vi "SwerveWheel.vi"(9 "rotate only?":bool, 10 "Inputs":dbl[](array[numeric]), 11 "Wheel":T1(ring)) -> (2 "Angle":dbl, 3 "Speed":dbl)   [LabVIEW 2019]
uses:
  <vilib>/Rock Robotics/WPI/ThirdParty/Phoenix-LabVIEW/Motor Controller/Controls/CTRE_Phoenix_MotorControl_ControlMode.ctl
  <vilib>/Analysis/coordinate.llb/Angle Range (Degree).ctl
  <vilib>/Analysis/coordinate.llb/Angle Units.ctl
  <vilib>/Analysis/coordinate.llb/Wrap Angle (scalar).vi
  Robot Global Data.vi
  <vilib>/Rock Robotics/WPI/ThirdParty/Phoenix-LabVIEW/Motor Controller/Get/CTRE_Phoenix_MotorController_IntegratedSensorData_TalonFX.vi
  <vilib>/Analysis/NI_AAL_Angle.lvlib
  <vilib>/Rock Robotics/WPI/ThirdParty/Phoenix-LabVIEW/Motor Controller/Controls/CTRE_Phoenix_MotorControl_TalonFXInvertType.ctl
  <vilib>/Rock Robotics/WPI/ThirdParty/Phoenix-LabVIEW/Motor Controller/Get/CTRE_Phoenix_MotorController_GetSupplyAndStatorCurrent_Enhanced.vi
  <vilib>/Rock Robotics/WPI/ThirdParty/Phoenix-LabVIEW/Motor Controller/Get/CTRE_Phoenix_MotorController_GetGeneralStatus.vi
panel:
  out "Z":bool
  out "Distance 2":dbl
  out "Distance":dbl
  out "Current Pos":dbl format="%.2f"
  out "Position to go to":dbl
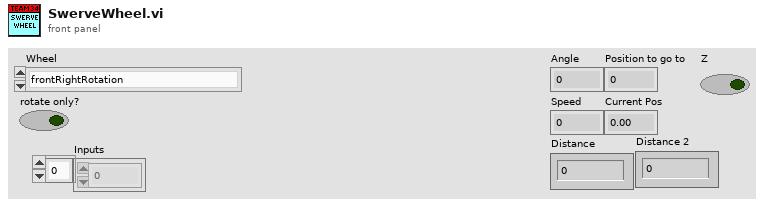
[diagram p1: front panel]
types:
  T1 = enum16{"frontRightRotation", "frontLeftRotation", "backRightRotation", "backLeftRotation"}
  T2 = typedef "NI_AAL_Angle.lvlib/Angle Units.ctl" = i32
  T3 = typedef "NI_AAL_Angle.lvlib/Angle Range (Degree).ctl" = u16
  T4 = typedef "CTRE_Phoenix_MotorControl_ControlMode.ctl" = u16
  T5 = typedef "CTRE_Phoenix_MotorControl_TalonFXInvertType.ctl" = enum16{"Counter-Clockwise", "Clockwise"}
  T6 = typedef "WPI_MotorControlDeviceRef.ctl" = cluster{"DeviceStatus":errorcluster, "Type":T7, "PWM":cluster{"PWM Channel":T8, "DeadBand":T9}, "CAN":cluster{"Device Number":u8, "SetOutput VI Ref":variant, "GetOutput VI Ref":variant, "Enable VI Ref":variant, "Disable VI Ref":variant, "Data":variant}, "Invert":bool, "DIO PWM":cluster{"PWM \"Enable\" Channel":T8, "DIOChannel":T10, "PWM Rate":dbl}}
  T7 = typedef "WPI_MotorControlType.ctl" = enum16{"PWM", "CAN", "DIO PWM"}
  T8 = typedef "FPGA_DIOPWMChannel.ctl" = enum8{"PWM 0", "PWM 1", "PWM 2", "PWM 3", "PWM 4", "PWM 5", "PWM 6", "PWM 7", "PWM 8", "PWM 9", "PWM MXP 0", "PWM MXP 1", "PWM MXP 2", "PWM MXP 3", "PWM MXP 4", "PWM MXP 5", "PWM MXP 6", "PWM MXP 7", "PWM MXP 8", "PWM MXP 9", "Invalid"}
  T9 = typedef "WPI_PWMDeadband.ctl" = cluster{"Name":string, "maxPositivePwm":i32, "minPositivePwm":i32, "centerPwm":i32, "maxNegativePwm":i32, "minNegativePwm":i32, "angularRange":u16}
  T10 = typedef "FPGA_DIOChannel.ctl" = enum8{"DIO 0", "DIO 1", "DIO 2", "DIO 3", "DIO 4", "DIO 5", "DIO 6", "DIO 7", "DIO 8", "DIO 9", "DIO MXP 0", "DIO MXP 1", "DIO MXP 2", "DIO MXP 3", "DIO MXP 4", "DIO MXP 5", "DIO MXP 6", "DIO MXP 7", "DIO MXP 8", "DIO MXP 9", "DIO MXP 10", "DIO MXP 11", "DIO MXP 12", "DIO MXP 13", "DIO MXP 14", "DIO MXP 15", "SPI Port CS1", "SPI Port CS2", "SPI Port CS3", "SPI Port MISO", "SPI Port MOSI", "Invalid"}
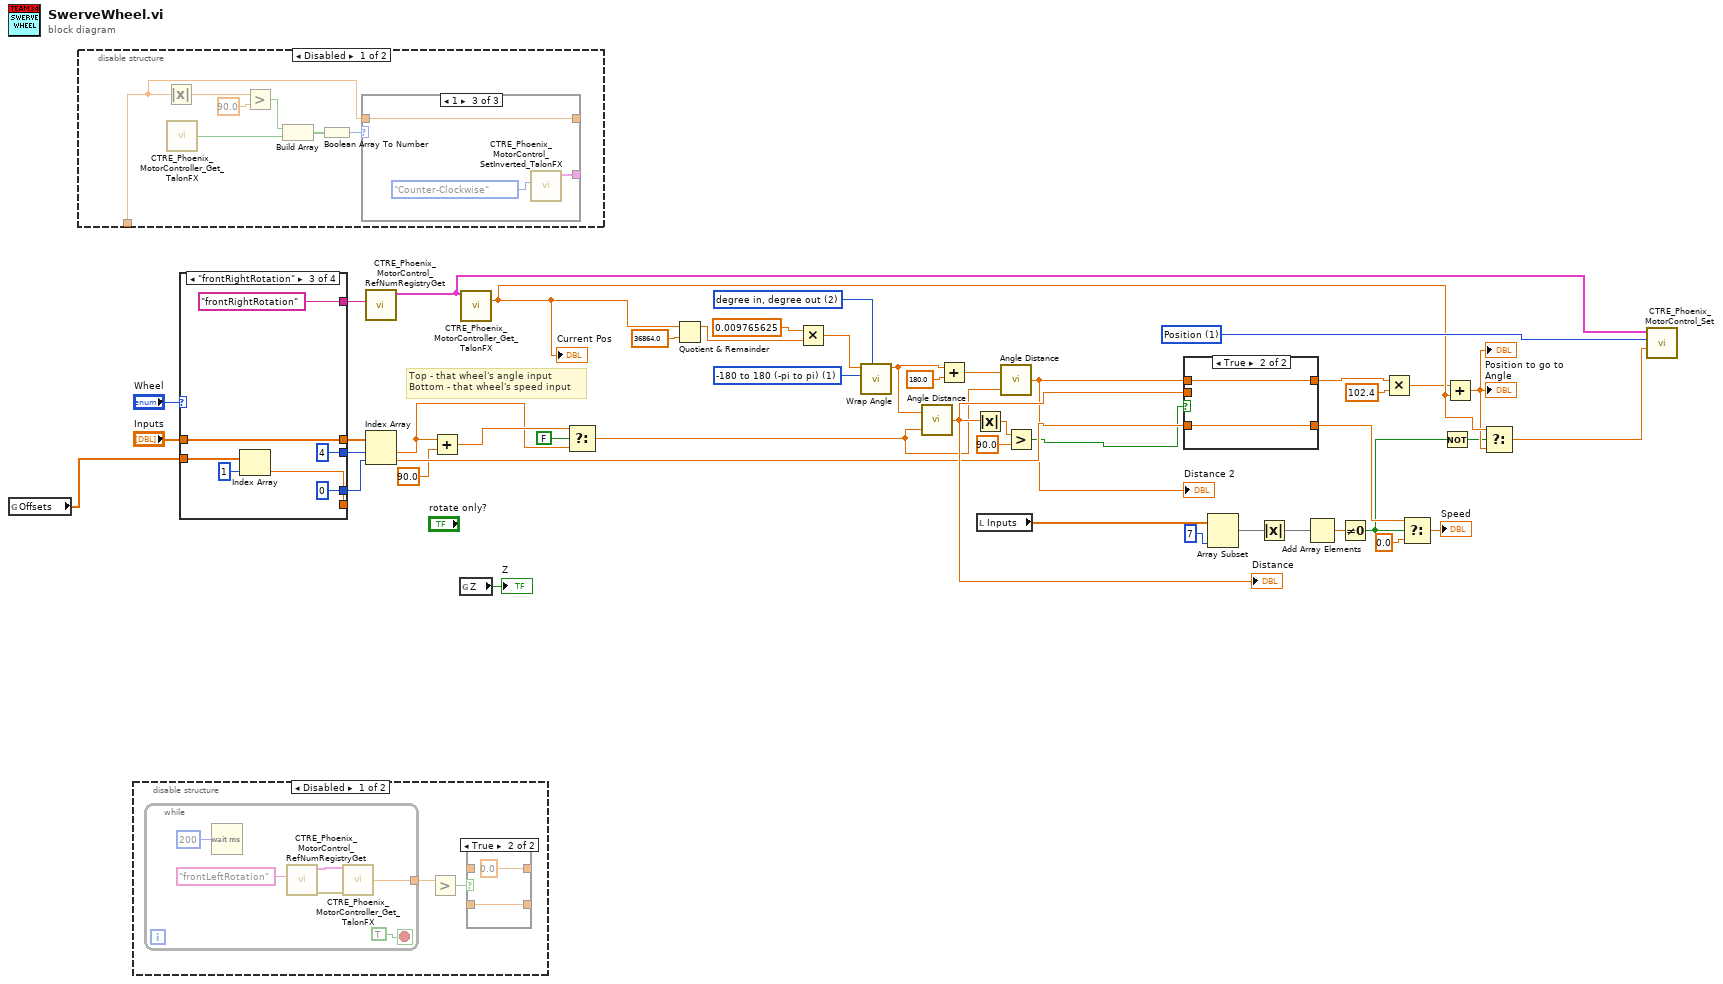
[diagram p0: block diagram]
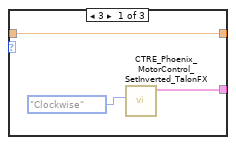
[diagram p2: hidden frame]
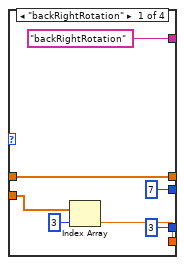
[diagram p5: hidden frame]
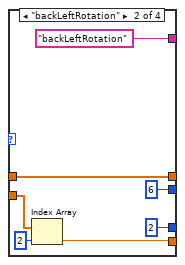
[diagram p6: hidden frame]
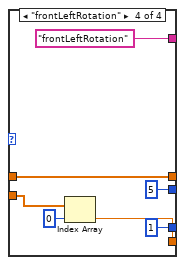
[diagram p7: hidden frame]
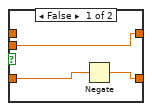
[diagram p10: hidden frame]
diagram:
  w43 = T2 2 items=["radian in, radian out", "radian in, degree out", "degree in, degree out", "degree in, radian out"] ("angle units")
  w44 = T3 1 items=["none", "-180 to 180 (-pi to pi)", "0 to 360 (0 to 2pi)"] ("angle range")
  w45 = T4 1 items=["PercentOutput"=0, "Position"=1, "Velocity"=2, "Current"=3, "Follower"=5, "MotionProfile"=6, "MotionMagic"=7, "MotionProfileArc"=10, "Disabled"=15] ("Control Mode")
  # "Top - that wheel's angle input\nBottom - that wheel's speed input"
  n1 = global read "Robot Global Data.vi" "Offsets"() -> (w10:dbl[])
  n2 = disable-structure shown="Disabled" {
    disable-tunnel: _ -> [w53 _]
    frame Disabled {
      n3 = Absolute Value(x=w53) -> (abs(x)=w52:dbl)
      n4 = call-poly <vilib>:"CTRE_Phoenix_MotorController_Get_TalonFX.vi"() -> ("Inverted?"=w49:bool)  [unwired: 10 in, 5 out]
      n5 = Greater?(x=w52, y=90.0) -> (0:w50:bool)
      n6 = Build Array(w50, w49) -> (w48:bool[])
      n7 = Boolean Array To Number(Boolean array=w48) -> (number=w47:u32)
      n8 = case shown="1" w47 {
        tunnel: w53 -> [w55 w57 w59]
        tunnel: [w55 w57 w59] -> _
        tunnel: [w54 _ w58] -> _
        frame 3 {
          n9 = call <vilib>:"CTRE_Phoenix_MotorControl_SetInverted_TalonFX.vi"("Invert Type"=CTRE_Phoenix_MotorControl_TalonFXInvertType."Clockwise") -> ("PhoenixMotorControlDevRef"=w54:T6)  [unwired: 9 in, 1 out]
        }
        frame 0, Default {
        }
        frame 1 {
          n10 = call <vilib>:"CTRE_Phoenix_MotorControl_SetInverted_TalonFX.vi"("Invert Type"=CTRE_Phoenix_MotorControl_TalonFXInvertType."Counter-Clockwise") -> ("PhoenixMotorControlDevRef"=w58:T6)  [unwired: 9 in, 1 out]
        }
      }
    }
    frame Enabled {
    }
  }
  n11 = disable-structure shown="Disabled" {
    frame Disabled {
      n12 = while {
        tunnel: [w67] -> w62
        stop <- TRUE stop-if-true
        n13 = Wait (ms)(milliseconds to wait=u32 200) -> ()  [unwired: 1 out]
        n14 = call <vilib>:"CTRE_Phoenix_MotorControl_RefNumRegistryGet.vi"("refnum name"="frontLeftRotation") -> ("error out"=w69:errorcluster, "PhoenixMotorControlDevRef"=w70:T6)  [unwired: 9 in]
        n15 = call-poly <vilib>:"CTRE_Phoenix_MotorController_Get_TalonFX.vi"("PhoenixMotorControlDevRef"=w70, "error in"=w69) -> ("Stator Current"=w67:dbl)  [unwired: 10 in, 3 out]
      }
      n16 = Greater?(x=w62) -> (0:w61:bool)  [unwired: 1 in]
      n17 = case shown="True" w61 {
        tunnel: [w64 0.0] -> _
        tunnel: _ -> [w64 _]
        tunnel: [w63 w66] -> _
        tunnel: _ -> [w63 w66]
        frame False {
        }
        frame True {
        }
      }
    }
    frame Enabled {
    }
  }
  n18 = case shown="\"frontRightRotation\"" "Wheel" {
    tunnel: ["backRightRotation" "backLeftRotation" "frontRightRotation" "frontLeftRotation"] -> w46
    tunnel: [3 ("index") 2 ("index") 0 ("index") 1 ("index")] -> w24
    tunnel: [7 ("index") 6 ("index") 4 ("index") 5 ("index")] -> w23
    tunnel: "Inputs" -> [w79 w86 w92 w97]
    tunnel: [w79 w86 w92 w97] -> w14
    tunnel: w10 -> [w75 w82 w89 w96]
    tunnel: [w74 w81 w88 w95] -> _
    frame "backRightRotation" {
      n19 = Index Array(array=w75, index=3) -> (element=w74:dbl)
    }
    frame "backLeftRotation" {
      n20 = Index Array(array=w82, index=2) -> (element=w81:dbl)
    }
    frame "frontRightRotation" {
      n21 = Index Array(array=w89, index=1) -> (element=w88:dbl)
    }
    frame "frontLeftRotation" {
      n22 = Index Array(array=w96, index=0) -> (element=w95:dbl)
    }
  }
  n23 = call <vilib>:"CTRE_Phoenix_MotorControl_RefNumRegistryGet.vi"("refnum name"=w46) -> ("PhoenixMotorControlDevRef"=w3:T6)  [unwired: 9 in, 1 out]
  n24 = Index Array(array=w14, index #1=w23, index #2=w24) -> (element #1=w5:dbl, element #2=w29:dbl)
  n25 = Add(x=w5, y=90.0) -> (x+y=w7:dbl)
  n26 = global read "Robot Global Data.vi" "Z"() -> (→"Z":bool)
  n27 = call-poly <vilib>:"CTRE_Phoenix_MotorController_Get_TalonFX.vi"("PhoenixMotorControlDevRef"=w3) -> ("Position"=w21:dbl)  [unwired: 10 in, 4 out]
  "Current Pos" <- w21
  n28 = Select(t=w7, s=FALSE, f=w5) -> (s? t:f=w6:dbl)
  n29 = Quotient & Remainder(x=w21, y=36864.0) -> (x-y*floor(x/y)=w26:dbl)  [unwired: 1 out]
  n30 = Multiply(x=0.009765625, y=w26) -> (x*y=w25:dbl)
  n31 = call-poly <vilib>:"Wrap Angle.vi"("angle units"=w43, "angle range"=w44, "angle in"=w25) -> ("angle out"=w40:dbl)  [unwired: 7 in, 1 out]
  n32 = call "Angle Distance.vi"("Target Angle"=w6, "Current Angle"=w40) -> ("Distance"=w39:dbl)
  "Distance" <- w39
  n33 = Add(x=w40, y=180.0) -> (x+y=w41:dbl)
  n34 = Absolute Value(x=w39) -> (abs(x)=w38:dbl)
  n35 = local read "Inputs"() -> (w31:dbl[])
  n36 = call "Angle Distance.vi"("Target Angle"=w6, "Current Angle"=w41) -> ("Distance"=w22:dbl)
  "Distance 2" <- w22
  n37 = Greater?(x=w38, y=90.0) -> (0:w8:bool)
  n38 = case shown="True" w8 {
    tunnel: w39 -> [w103 _]
    tunnel: w22 -> [_ w105]
    tunnel: [w102 w104] -> w19
    tunnel: [w103 w105] -> w2
    tunnel: w29 -> [w101 w104]
    frame False {
      n39 = Negate(x=w101) -> (-x=w102:dbl)
    }
    frame True {
    }
  }
  n40 = Array Subset(array=w31, length=7) -> (w33:dbl[])  [unwired: 1 in]
  n41 = Absolute Value(x=w33) -> (abs(x)=w34:dbl[])
  n42 = Add Array Elements(numeric array=w34) -> (sum=w32:dbl)
  n43 = Not Equal To 0?(x=w32) -> (x != 0?=w17:bool)
  n44 = Multiply(x=w2, y=102.4) -> (x*y=w11:dbl)
  n45 = Select(t=w19, s=w17, f=0.0) -> (s? t:f=→"Speed":dbl)
  n46 = Not(x=w17) -> (.not. x?=w18:bool)
  n47 = Add(x=w11, y=w21) -> (x+y=w20:dbl)
  "Angle" <- w20
  "Position to go to" <- w20
  n48 = Select(t=w21, s=w18, f=w20) -> (s? t:f=w16:dbl)
  n49 = call <vilib>:"CTRE_Phoenix_MotorControl_Set.vi"("Output"=w16, "Control Mode"=w45, "PhoenixMotorControlDevRef"=w3) -> ()  [unwired: 7 in, 2 out]
